vi "ResetGlobalVariables.vi"   [LabVIEW 2020]
doc: "This VI sets non-robot specific constants and initializes critical global variables."
uses:
  robotconstants.vi
  robotoutputs.vi
  sensordata.vi
  drivercommands.vi
  driverdata.vi
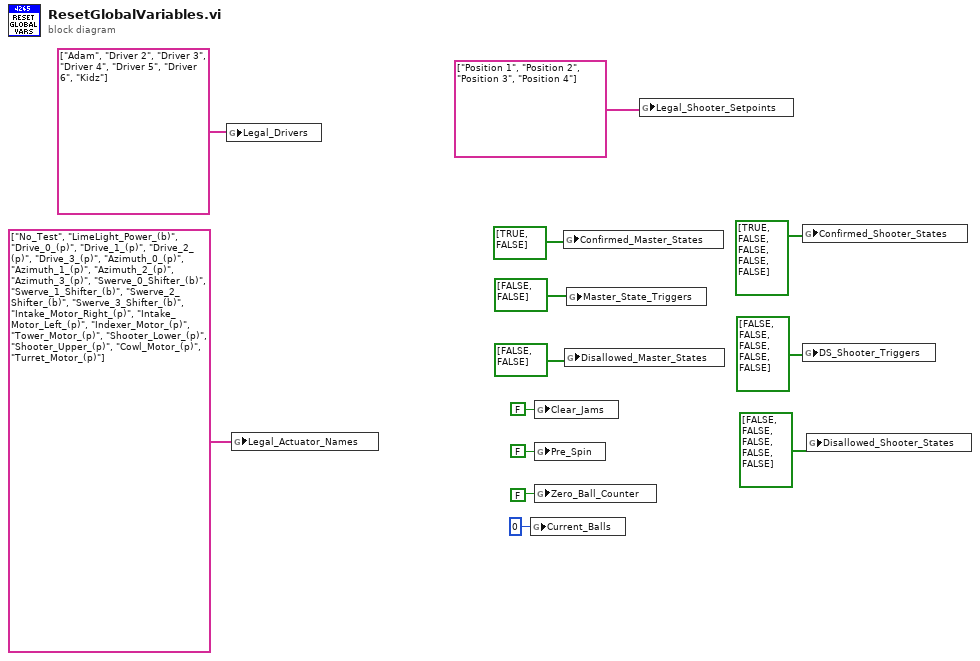
[diagram p0: block diagram]
diagram:
  n1 = global write "robotconstants.vi" "Legal_Drivers"(string[] ["Adam", "Driver 2", "Driver 3", "Driver 4", "Driver 5", "Driver 6", "Kidz"] ("appended array")) -> ()
  n2 = global write "robotconstants.vi" "Legal_Actuator_Names"(string[] ["No_Test", "LimeLight_Power_(b)", "Drive_0_(p)", "Drive_1_(p)", "Drive_2_(p)", "Drive_3_(p)", "Azimuth_0_(p)", "Azimuth_1_(p)", "Azimuth_2_(p)", "Azimuth_3_(p)", "Swerve_0_Shifter_(b)", "Swerve_1_Shifter_(b)", "Swerve_2_Shifter_(b)", "Swerve_3_Shifter_(b)", "Intake_Motor_Right_(p)", "Intake_Motor_Left_(p)", "Indexer_Motor_(p)", "Tower_Motor_(p)", "Shooter_Lower_(p)", "Shooter_Upper_(p)", "Cowl_Motor_(p)", "Turret_Motor_(p)"] ("appended array")) -> ()
  n3 = global write "sensordata.vi" "Current_Balls"(0 ("Current_Balls")) -> ()
  n4 = global write "drivercommands.vi" "Clear_Jams"(FALSE ("Clear_Jams")) -> ()
  n5 = global write "drivercommands.vi" "Pre_Spin"(FALSE ("Pre_Spin")) -> ()
  n6 = global write "driverdata.vi" "Zero_Ball_Counter"(FALSE ("Zero_Ball_Counter")) -> ()
  n7 = global write "robotoutputs.vi" "Confirmed_Master_States"(bool[] [TRUE, FALSE] ("Disallowed_Master_States")) -> ()
  n8 = global write "robotoutputs.vi" "Disallowed_Master_States"(bool[] [FALSE, FALSE] ("Disallowed_Master_States")) -> ()
  n9 = global write "drivercommands.vi" "Master_State_Triggers"(bool[] [FALSE, FALSE] ("Disallowed_Master_States")) -> ()
  n10 = global write "robotconstants.vi" "Legal_Shooter_Setpoints"(string[] ["Position 1", "Position 2", "Position 3", "Position 4"] ("appended array")) -> ()
  n11 = global write "robotoutputs.vi" "Confirmed_Shooter_States"(bool[] [TRUE, FALSE, FALSE, FALSE, FALSE] ("Disallowed_Master_States")) -> ()
  n12 = global write "drivercommands.vi" "DS_Shooter_Triggers"(bool[] [FALSE, FALSE, FALSE, FALSE, FALSE] ("Disallowed_Master_States")) -> ()
  n13 = global write "robotoutputs.vi" "Disallowed_Shooter_States"(bool[] [FALSE, FALSE, FALSE, FALSE, FALSE] ("Disallowed_Master_States")) -> ()
